vi "__AttrMap-GetValue2.vi"(8 "error in (no error)":errorcluster, 9 "Key":string, 11 "AttrMap in":T1) -> (0 "error out":errorcluster, 1 "found":bool, 2 "VAttributes":variant, 3 "AttrMap out":T1, 4 "OrignKey":string)   [LabVIEW 2019, in "lv-apt-json-file.lvlib"]
uses:
  lv-apt-json-file.lvlib
  Typedef/Def-AttrMap.ctl
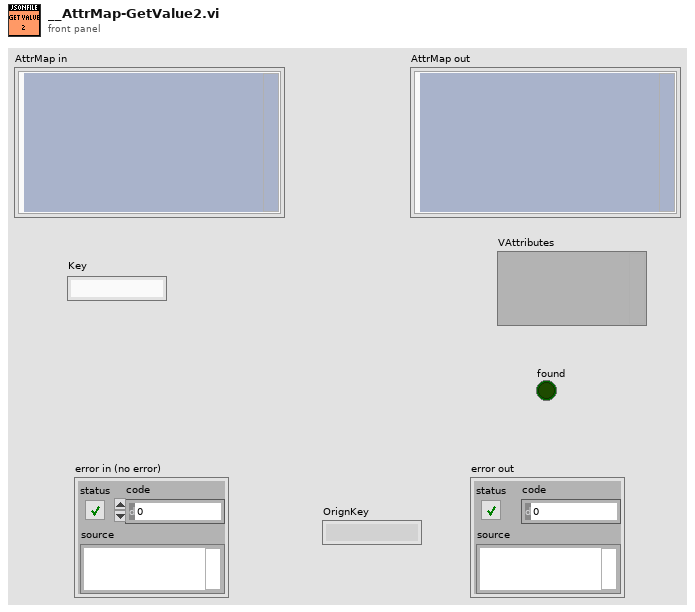
[diagram p1: front panel]
types:
  T1 = typedef "lv-apt-json-file.lvlib/Def-AttrMap.ctl" = cluster{"Map":variant}
  T2 = typedef "lv-apt-json-file.lvlib/Def-NameMap.ctl" = variant[]
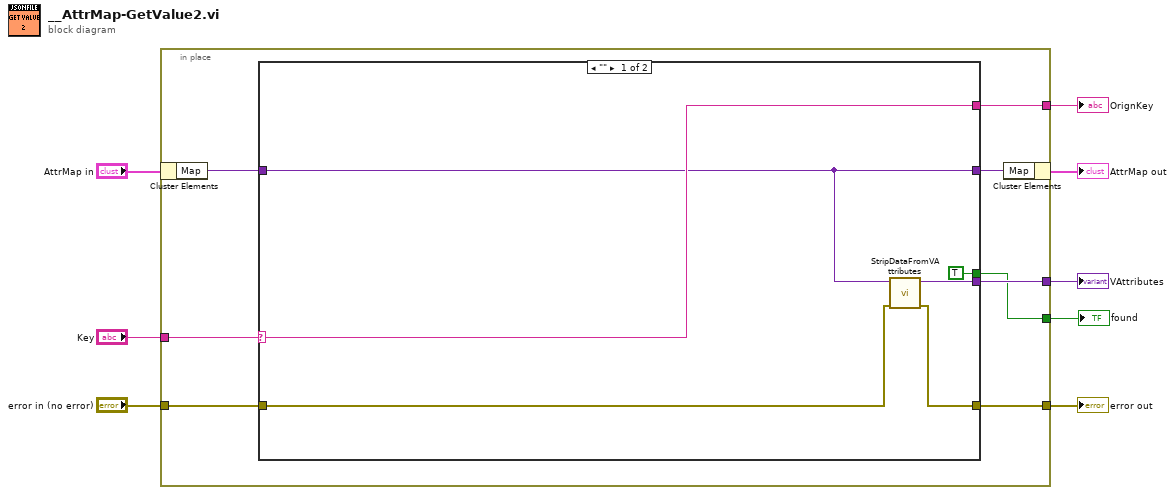
[diagram p0: block diagram]
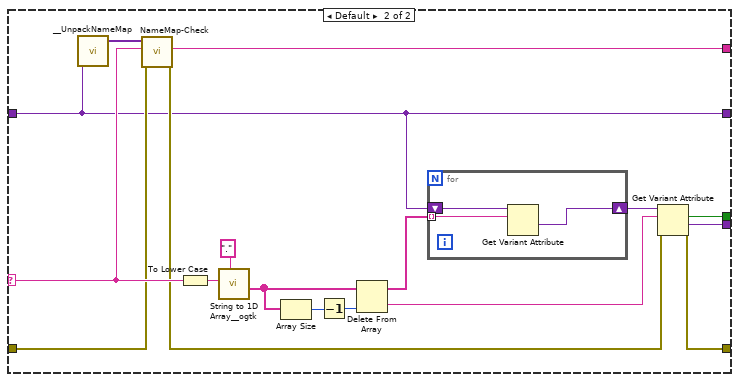
[diagram p2: hidden frame]
diagram:
  n1 = in-place "In Place Element Structure" {
    in-place-border: [w12] -> w8
    in-place-border: "error in (no error)" -> [w14]
    in-place-border: "Key" -> [w15]
    in-place-border: [w13] -> w3
    in-place-border: [w11] -> w2
    in-place-border: [w10] -> w1
    n2 = in-place-cluster #1("AttrMap in") -> ("Map"=w16:variant)
    n3 = case shown="\"\"" w15 {
      selector: w15 -> [w22 w30]
      tunnel: w16 -> [w21 w23]
      tunnel: w14 -> [w18 w29]
      tunnel: [w19 w27] -> w13
      tunnel: [w17 w26] -> w12
      tunnel: [w22 w25] -> w11
      tunnel: [TRUE w24] -> w10
      tunnel: [w21 w23] -> w9
      frame "" {
        n4 = call "StripDataFromVAttributes.vi"("error in (no error)"=w18, "Map"=w21) -> ("error out"=w17:errorcluster, "duplicate variant"=w19:variant)  [unwired: 8 in]
      }
      frame Default {
        n5 = call "__UnpackNameMap.vi"("Map"=w23) -> ("NameMap"=w31:T2)  [unwired: 10 in]
        n6 = call "NameMap-Check.vi"("error in (no error)"=w29, "Name"=w30, "NameMap in"=w31) -> ("error out"=w28:errorcluster, "OriginName"=w25:string)  [unwired: 6 in, 1 out]
        n7 = To Lower Case(string=w30) -> (all lower case string=w37:string)
        n8 = call <userlib>:"String to 1D Array__ogtk.vi"("delimiter (Tab)"=".", "string"=w37) -> ("Array of Strings"=w34:string[])  [unwired: 9 in]
        n9 = Array Size(array=w34) -> (size(s)=w38:i32)
        n10 = Decrement(x=w38) -> (x-1=w32:i32)
        n11 = Delete From Array(array=w34, index=w32) -> (deleted portion=w35:string, array with subset deleted=w33:string[])  [unwired: 1 in]
        n12 = for {
          tunnel: w33 -> [w41] mode=indexing
          shift-right: [w40] -> w36
          shift-left: w23 -> [w42]
          n13 = Get Variant Attribute(Variant=w42, name=w41) -> (value=w40:variant)  [unwired: 2 in, 3 out]
        }
        n14 = Get Variant Attribute(Variant=w36, name=w35, error in=w28) -> (found=w24:bool, value=w27:variant, error out=w26:errorcluster)  [unwired: 1 in, 1 out]
      }
    }
    n15 = in-place-cluster #1("Map"=w9) -> (→"AttrMap out":T1)
  }
  "error out" <- w8
  "VAttributes" <- w3
  "OrignKey" <- w2
  "found" <- w1
